vi "Clappy up down.vi"(0 "UP/Down":dbl, 1 "UP DOWN ENCODER":T9={"DevStatus"={"status"=FALSE, "code"=0, "source"=""}, "EncoderIndex"=enum."Invalid", "CounterIndex"=enum."Ctr 1", "DistancePerCount"=2.0, "Decoding Type"=enum."4x"}, 2 "UPDOWN":T1={"DeviceStatus"={"status"=FALSE, "code"=0, "source"=""}, "Type"=enum."PWM", "PWM"={"PWM Channel"=enum."Invalid", "DeadBand"={"Name"="", "maxPositivePwm"=0, "minPositivePwm"=0, "centerPwm"=0, "maxNegativePwm"=0, "minNegativePwm"=0, "angularRange"=0}}, "CAN"={"Device Number"=0, "Control Mode"=enum."Percent VBus", "Semaphore"=refnum, "Max Vout"=12.0, "TalonSRX Control Mode"=enum."Percent VBus"}, "Invert"=FALSE}, 3 "Manual":bool, 5 "Negate 1":bool, 7 "Open/Closed 1":dbl, 9 "Negate 2":bool, 11 "Open/Closed 2":dbl, 12 "Clappy":T8={"DevStatus"={"status"=FALSE, "code"=0, "source"=""}, "Motors[]"=[], "Square Inputs"=FALSE, "Max Output"=1.0}, 13 "OPEN CLOSED ENCODER 1":T9={"DevStatus"={"status"=FALSE, "code"=0, "source"=""}, "EncoderIndex"=enum."Invalid", "CounterIndex"=enum."Ctr 1", "DistancePerCount"=2.0, "Decoding Type"=enum."4x"}, 14 "OPEN CLOSED ENCODER 2":T9={"DevStatus"={"status"=FALSE, "code"=0, "source"=""}, "EncoderIndex"=enum."Invalid", "CounterIndex"=enum."Ctr 1", "DistancePerCount"=2.0, "Decoding Type"=enum."4x"}) -> ()   [LabVIEW 2015]
uses:
  <vilib>/Rock Robotics/WPI/Encoder/WPI_EncoderDevRef.ctl
  <vilib>/Rock Robotics/SystemInterfaces/Encoder/FPGA_EncoderIdx.ctl
  <vilib>/Rock Robotics/SystemInterfaces/Counter/FPGA_CounterCtrSystemIndex.ctl
  <vilib>/Rock Robotics/WPI/Encoder/WPI_EncoderType.ctl
  <vilib>/Rock Robotics/WPI/RobotDrive/WPI_RobotDriveDevRef.ctl
  <vilib>/Rock Robotics/WPI/MotorControl/WPI_MotorControlDeviceRef.ctl
  <vilib>/Rock Robotics/WPI/MotorControl/WPI_MotorControlType.ctl
  <vilib>/Rock Robotics/SystemInterfaces/DIO/FPGA_DIOPWMChannel.ctl
  <vilib>/Rock Robotics/WPI/PWM/WPI_PWMDeadband.ctl
  <vilib>/Rock Robotics/WPI/CAN/Jaguar/SubVIs/WPI_CANJaguar_ControlMode.ctl
  <vilib>/Rock Robotics/WPI/CAN/TalonSRX/WPI_CANTalonSRX_APIControlMode.ctl
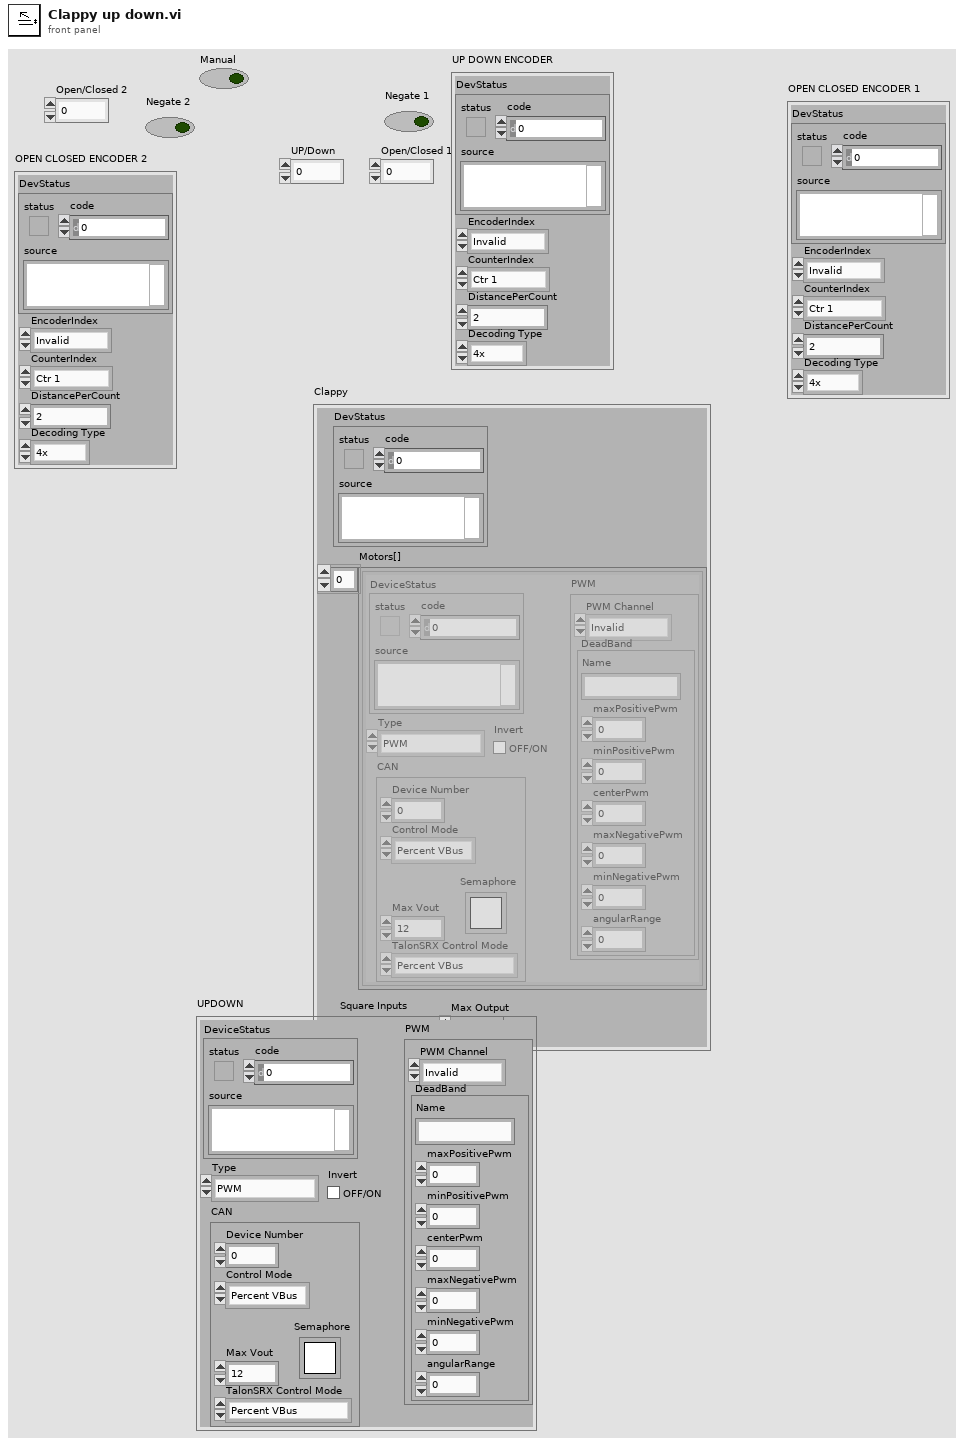
[diagram p1: front panel]
types:
  T1 = typedef "WPI_MotorControlDeviceRef.ctl" = cluster{"DeviceStatus":errorcluster, "Type":T2, "PWM":cluster{"PWM Channel":T3, "DeadBand":T4}, "CAN":cluster{"Device Number":u8, "Control Mode":T5, "Semaphore":T6, "Max Vout":dbl, "TalonSRX Control Mode":T7}, "Invert":bool}
  T2 = typedef "WPI_MotorControlType.ctl" = enum16{"PWM", "CAN", "CANTalonSRX"}
  T3 = typedef "FPGA_DIOPWMChannel.ctl" = enum8{"PWM 0", "PWM 1", "PWM 2", "PWM 3", "PWM 4", "PWM 5", "PWM 6", "PWM 7", "PWM 8", "PWM 9", "PWM MXP 0", "PWM MXP 1", "PWM MXP 2", "PWM MXP 3", "PWM MXP 4", "PWM MXP 5", "PWM MXP 6", "PWM MXP 7", "PWM MXP 8", "PWM MXP 9", "Invalid"}
  T4 = typedef "WPI_PWMDeadband.ctl" = cluster{"Name":string, "maxPositivePwm":i32, "minPositivePwm":i32, "centerPwm":i32, "maxNegativePwm":i32, "minNegativePwm":i32, "angularRange":u16}
  T5 = typedef "WPI_CANJaguar_ControlMode.ctl" = enum8{"Percent VBus", "Current", "Speed", "Position", "Voltage"}
  T6 = typedef "Semaphore RefNum" = refnum<k1>
  T7 = typedef "WPI_CANTalonSRX_APIControlMode.ctl" = enum8{"Percent VBus", "Speed", "Position", "Slave", "Unchanged / Invalid", "Voltage Compensation", "Current", "Motion Profile"}
  T8 = typedef "WPI_RobotDriveDevRef.ctl" = cluster{"DevStatus":errorcluster, "Motors[]":T1[], "Square Inputs":bool, "Max Output":dbl}
  T9 = typedef "WPI_EncoderDevRef.ctl" = cluster{"DevStatus":errorcluster, "EncoderIndex":T10, "CounterIndex":T11, "DistancePerCount":dbl, "Decoding Type":T12}
  T10 = typedef "FPGA_EncoderIdx.ctl" = enum8{"Enc 0", "Enc 1", "Enc 2", "Enc 3", "Enc 4", "Enc 5", "Enc 6", "Enc 7", "Invalid"}
  T11 = typedef "FPGA_CounterCtrSystemIndex.ctl" = enum8{"Ctr 0", "Ctr 1", "Ctr 2", "Ctr 3", "Ctr 4", "Ctr 5", "Ctr 6", "Ctr 7", "Invalid"}
  T12 = typedef "WPI_EncoderType.ctl" = enum16{"1x", "2x", "4x"}
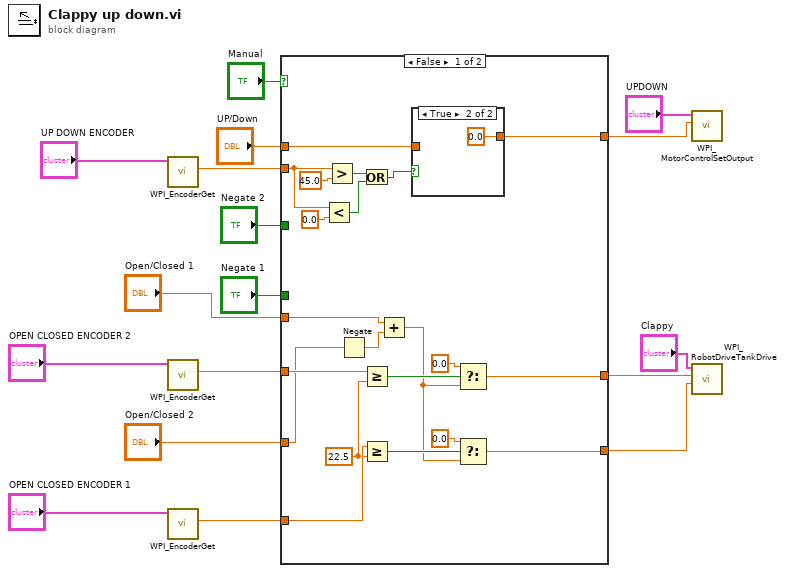
[diagram p0: block diagram]
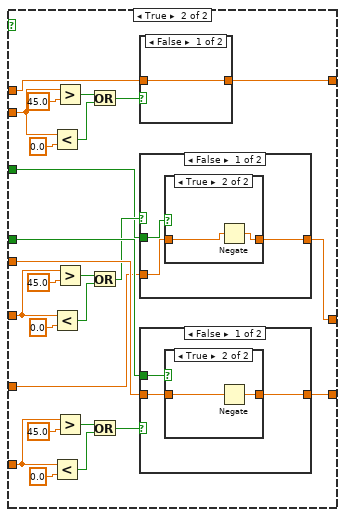
[diagram p3: hidden frame]
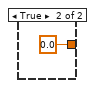
[diagram p5: hidden frame]
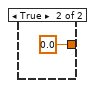
[diagram p7: hidden frame]
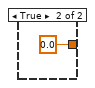
[diagram p8: hidden frame]
diagram:
  n1 = call <vilib>:"WPI_EncoderGet.vi"("EncoderDevRef"="UP DOWN ENCODER") -> ("Distance"=w10:dbl)  [unwired: 5 in, 5 out]
  n2 = call <vilib>:"WPI_EncoderGet.vi"("EncoderDevRef"="OPEN CLOSED ENCODER 2") -> ("Distance"=w8:dbl)  [unwired: 5 in, 5 out]
  n3 = call <vilib>:"WPI_EncoderGet.vi"("EncoderDevRef"="OPEN CLOSED ENCODER 1") -> ("Distance"=w12:dbl)  [unwired: 5 in, 5 out]
  n4 = case shown="False" "Manual" {
    tunnel: "Open/Closed 1" -> [w18 w51]
    tunnel: "UP/Down" -> [w23 w64]
    tunnel: "Negate 1" -> [_ w52]
    tunnel: [w22 w65] -> w4
    tunnel: [w35 w50] -> w6
    tunnel: w12 -> [w36 w53]
    tunnel: w10 -> [w24 w60]
    tunnel: w8 -> [w34 w42]
    tunnel: [w30 w41] -> w7
    tunnel: "Negate 2" -> [_ w44]
    tunnel: "Open/Closed 2" -> [w19 w43]
    frame False {
      w33 = 22.5 ("y")
      n5 = Less?(x=w24, y=0.0) -> (x < y?=w27:bool)
      n6 = Greater?(x=w24, y=45.0) -> (0:w28:bool)
      n7 = Negate(x=w19) -> (-x=w21:dbl)
      n8 = Or(x=w28, y=w27) -> (x .or. y?=w26:bool)
      n9 = Greater Or Equal?(x=w34, y=w33) -> (x >= y?=w31:bool)
      n10 = Greater Or Equal?(x=w36, y=w33) -> (x >= y?=w38:bool)
      n11 = Add(x=w18, y=w21) -> (x+y=w20:dbl)
      n12 = case shown="True" w26 {
        tunnel: [w39 0.0 ("UP/Down")] -> w22
        tunnel: w23 -> [w39 _]
        frame False {
        }
        frame True {
        }
      }
      n13 = Select(t=0.0, s=w31, f=w20) -> (s? t:f=w30:dbl)
      n14 = Select(t=0.0, s=w38, f=w20) -> (s? t:f=w35:dbl)
    }
    frame True {
      n15 = Less?(x=w60, y=0.0) -> (x < y?=w62:bool)
      n16 = Less?(x=w42, y=0.0) -> (x < y?=w47:bool)
      n17 = Less?(x=w53, y=0.0) -> (x < y?=w56:bool)
      n18 = Greater?(x=w60, y=45.0) -> (0:w63:bool)
      n19 = Greater?(x=w42, y=45.0) -> (0:w46:bool)
      n20 = Greater?(x=w53, y=45.0) -> (0:w57:bool)
      n21 = Or(x=w63, y=w62) -> (x .or. y?=w61:bool)
      n22 = Or(x=w46, y=w47) -> (x .or. y?=w48:bool)
      n23 = Or(x=w57, y=w56) -> (x .or. y?=w55:bool)
      n24 = case shown="False" w61 {
        tunnel: [w81 0.0 ("UP/Down")] -> w65
        tunnel: w64 -> [w81 _]
        frame False {
        }
        frame True {
        }
      }
      n25 = case shown="False" w48 {
        tunnel: [w68 0.0 ("UP/Down")] -> w41
        tunnel: w44 -> [w69 _]
        tunnel: w43 -> [w67 _]
        frame False {
          n26 = case shown="True" w69 {
            tunnel: [w70 w72] -> w68
            tunnel: w67 -> [w70 w71]
            frame False {
            }
            frame True {
              n27 = Negate(x=w71) -> (-x=w72:dbl)
            }
          }
        }
        frame True {
        }
      }
      n28 = case shown="False" w55 {
        tunnel: [w74 0.0 ("UP/Down")] -> w50
        tunnel: w52 -> [w76 _]
        tunnel: w51 -> [w75 _]
        frame False {
          n29 = case shown="True" w76 {
            tunnel: w75 -> [w77 w79]
            tunnel: [w77 w78] -> w74
            frame False {
            }
            frame True {
              n30 = Negate(x=w79) -> (-x=w78:dbl)
            }
          }
        }
        frame True {
        }
      }
    }
  }
  n31 = call <vilib>:"WPI_MotorControlSetOutput.vi"("Output"=w4, "MotorControlDevRef"="UPDOWN") -> ()  [unwired: 7 in, 3 out]
  n32 = call <vilib>:"WPI_RobotDriveTankDrive.vi"("Right axis value"=w6, "Left axis value"=w7, "RobotDriveDevRef"="Clappy") -> ()  [unwired: 6 in, 3 out]
